vi "Cal Days of Month.vi"(5 "date":cluster{"year":u16, "month":u16}) -> (2 "days":u16)   [LabVIEW 2020]
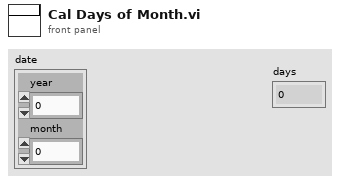
[diagram p1: front panel]
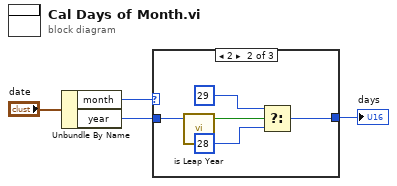
[diagram p0: block diagram]
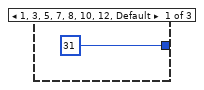
[diagram p2: hidden frame]
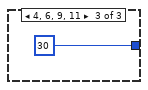
[diagram p3: hidden frame]
diagram:
  n1 = Unbundle By Name("date") -> ("month"=w2:u16, "year"=w1:u16)
  n2 = case shown="2" w2 {
    tunnel: [u16 31 ("days") w6 u16 30 ("days")] -> w4
    tunnel: w1 -> [_ w10 _]
    frame 1, 3, 5, 7, 8, 10, 12, Default {
    }
    frame 2 {
      n3 = call "is Leap Year.vi"("year"=w10) -> ("lear year?"=w9:bool)  [unwired: 4 in]
      n4 = Select(t=u16 29 ("days"), s=w9, f=u16 28 ("days")) -> (s? t:f=w6:u16)
    }
    frame 4, 6, 9, 11 {
    }
  }
  "days" <- w4
